vi "L1ManualControl.vi"() -> ()   [LabVIEW 2012]
uses:
  <vilib>/Utility/NIReport.llb/NI_report.lvclass
  <vilib>/Utility/NIReport.llb/HTML/NI_HTML.lvclass
panel:
  out "data read value":u32=36
  out "data out serial":string="0_2-63@36\r\n"
  in  "Data":i32
  in  "Register or channel":i32=96
  in  "RD/#WR":bool
  in  "Combination":i32 min=0 max=127 step=1 format="%b"
  in  "Voltage Input":dbl(slide)=0.33316326530612245 scale=0.05..0.8
  in  "Amp Scaler":dbl(slide)=0.1 scale=0.1..10.0
  in  "stop":bool
  in  "Single Channel Enable":i32(slide) scale=0.0..6.0
  in  "Single/Comb":bool=TRUE
  out "error out":errorcluster
  in  "Instrument VISA in":T1={"AWG VISA"="AgilentGenerator1", "Oscilloscope  VISA "="AgilentOsciloscope", "Integration Board IP"="172.16.7.47", "connection ID"=refnum, "report out"=refnum, "report file path"=path "C:/Documents and Settings/CTA_LAB01/Desktop/L0_Asic/L0 Asic Test Data"}
  in  "error in (no error)":errorcluster
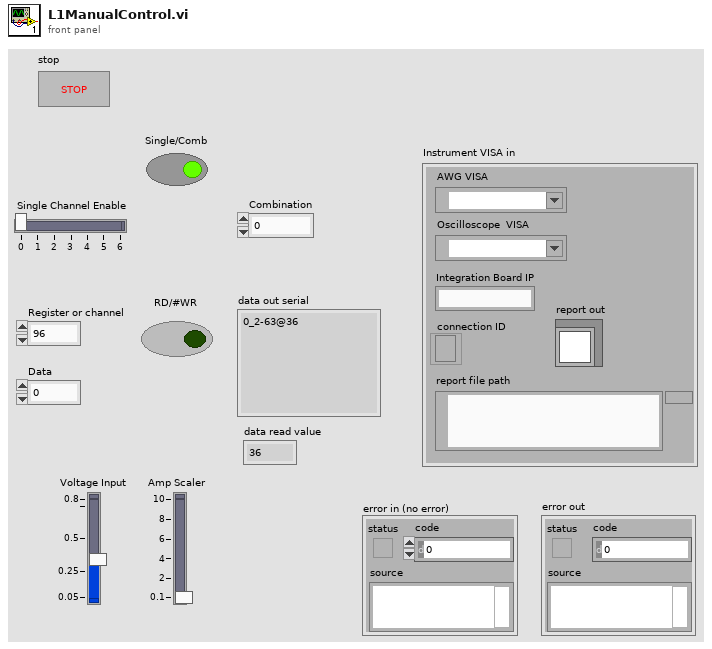
[diagram p1: front panel]
types:
  T1 = cluster{"AWG VISA":refnum<visa-resource-name>, "Oscilloscope  VISA ":refnum<visa-resource-name>, "Integration Board IP":string, "connection ID":refnum<k5>, "report out":refnum<class "NI_report.lvclass">, "report file path":path}
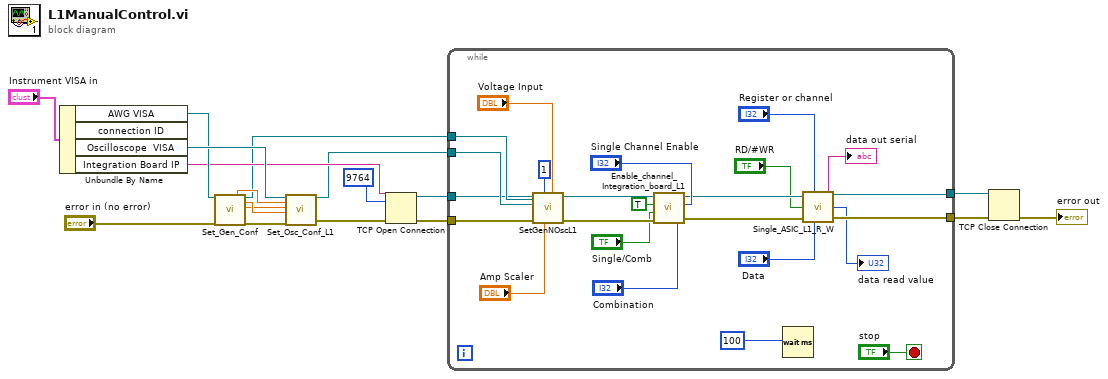
[diagram p0: block diagram]
diagram:
  n1 = Unbundle By Name("Instrument VISA in") -> ("AWG VISA"=w14:refnum<visa-resource-name>, "Oscilloscope  VISA"=w15:refnum<visa-resource-name>, "Integration Board IP"=w9:string)  [unwired: 1 out]
  n2 = call "Set_Gen_Conf.vi"("AWG VISA"=w14, "error in (no error)"="error in (no error)") -> ("Amplitude 1 OUT"=w12:dbl, "VISA resource name out"=w5:refnum<visa-resource-name>, "Pulse Width in seconds 1 OUT"=w11:dbl, "Trigger Level 1"=w10:dbl, "error out"=w17:errorcluster)  [unwired: 10 in, 3 out]
  n3 = call "Set_Osc_Conf_L1.vi"("VISA resource name"=w15, "Amplitude IN"=w12, "Trigger Level IN"=w10, "Pulse Width in seconds IN"=w11, "error in (no error)"=w17) -> ("VISA resource name out"=w4:refnum<visa-resource-name>, "error out"=w1:errorcluster)  [unwired: 13 in]
  n4 = TCP Open Connection(address=w9, remote port or service name=9764, error in (no error)=w1) -> (connection ID=w3:refnum<k5>, error out=w2:errorcluster)  [unwired: 2 in]
  n5 = while {
    tunnel: [w25] -> w7
    tunnel: [w24] -> w6
    tunnel: w4 -> [w41]
    tunnel: w5 -> [w40]
    tunnel: w2 -> [w39]
    tunnel: w3 -> [w32]
    stop <- "stop" stop-if-true
    n6 = call "SetGenNOscL1.vi"("Input Voltage"="Voltage Input", "Amp Scaler"="Amp Scaler", "NChannels"=1, "error in (no error)"=w39, "VISA resource name"=w41, "AWG VISA"=w40) -> ("error out 2"=w33:errorcluster)  [unwired: 5 in]
    n7 = call "Enable_channel_Integration_board_L1.vi"("Cobination"="Combination", "Enable  L1 single  Input"="Single Channel Enable", "error in (no error)"=w33, "SingleIN/#Combination"="Single/Comb", "#Enable all L1"=TRUE, "connection ID"=w32) -> ("error out"=w27:errorcluster, "connection ID out"=w26:refnum<k5>)
    n8 = Wait (ms)(milliseconds to wait=100) -> ()  [unwired: 1 out]
    n9 = call "Single_ASIC_L1_R_W.vi"("connection ID"=w26, "Register or channel"="Register or channel", "RD/#WR"="RD/#WR", "error in (no error)"=w27, "Data"="Data") -> ("data out serial"=→"data out serial":string, "connection ID out"=w24:refnum<k5>, "data read value"=→"data read value":u32, "error out"=w25:errorcluster)  [unwired: 1 in]
  }
  n10 = TCP Close Connection(connection ID=w6, error in (no error)=w7) -> (error out=→"error out":errorcluster)  [unwired: 1 in, 1 out]
